vi "Async Test With Results.vi"() -> ()   [LabVIEW 2015, in "ResultProcessor Tests.lvlib"]
uses:
  ResultProcessor Tests.lvlib
  Report Information/DUT Information.ctl
  Report Information/Station Information.ctl
  Report Information/Test Information.ctl
  Execution/ResultProcessor.lvclass
  Config/ResultProcessor Config.lvclass
  Report/On-The-Fly/Config/OnTheFlyReport Config.lvclass
  Report Formatters/csv/Config/csv-formatter Config.lvclass
  Result/Result.lvclass
  Report Information/Report Information.lvclass
panel:
  in  "Report Path":path
  in  "stop":bool
  in  "Measurement":string
  in  "Low Limit":string
  in  "High Limit":string
  in  "Duration (ms)":dbl
  in  "Step Class":string
  in  "Comparison Type":string
  in  "Step Name":string
  in  "Publish Report":bool
  in  "New Report":bool
  in  "Add Result":bool
  in  "Add Test Info":bool
  in  "Add Station Info":bool
  in  "Add DUT Info":bool
  in  "Test Information":T1
  in  "Station Info":T2
  in  "DUT Info":T3
  out "AsyncWorkerError":errorcluster
  out "error out":errorcluster
  # "Run the VI\nPick a file name. Can be an empty file or a new file name.\nSelect New Report\nData entered in the various fields will be sent to the processor each time you press the cooresponding button"
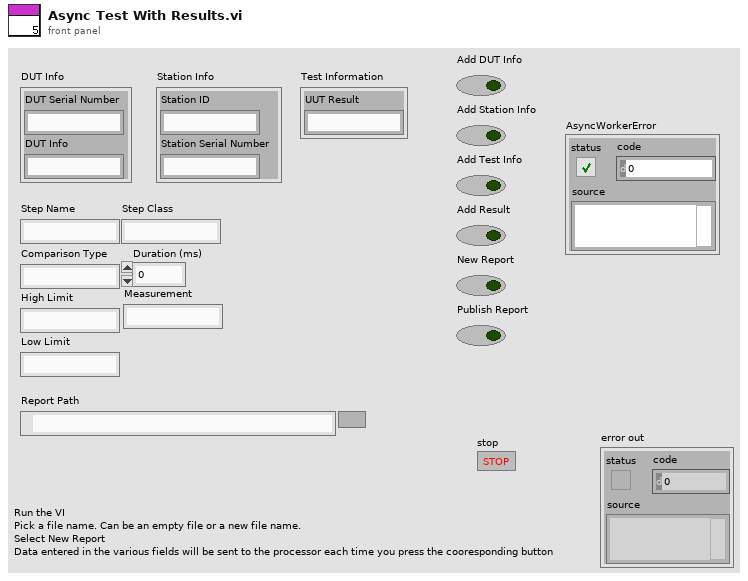
[diagram p1: front panel]
types:
  T1 = typedef "Report Information.lvclass/Test Information.ctl" = cluster{"UUT Result":string}
  T2 = typedef "Report Information.lvclass/Station Information.ctl" = cluster{"Station ID":string, "Station Serial Number":string}
  T3 = typedef "Report Information.lvclass/DUT Information.ctl" = cluster{"DUT Serial Number":string, "DUT Info":string}
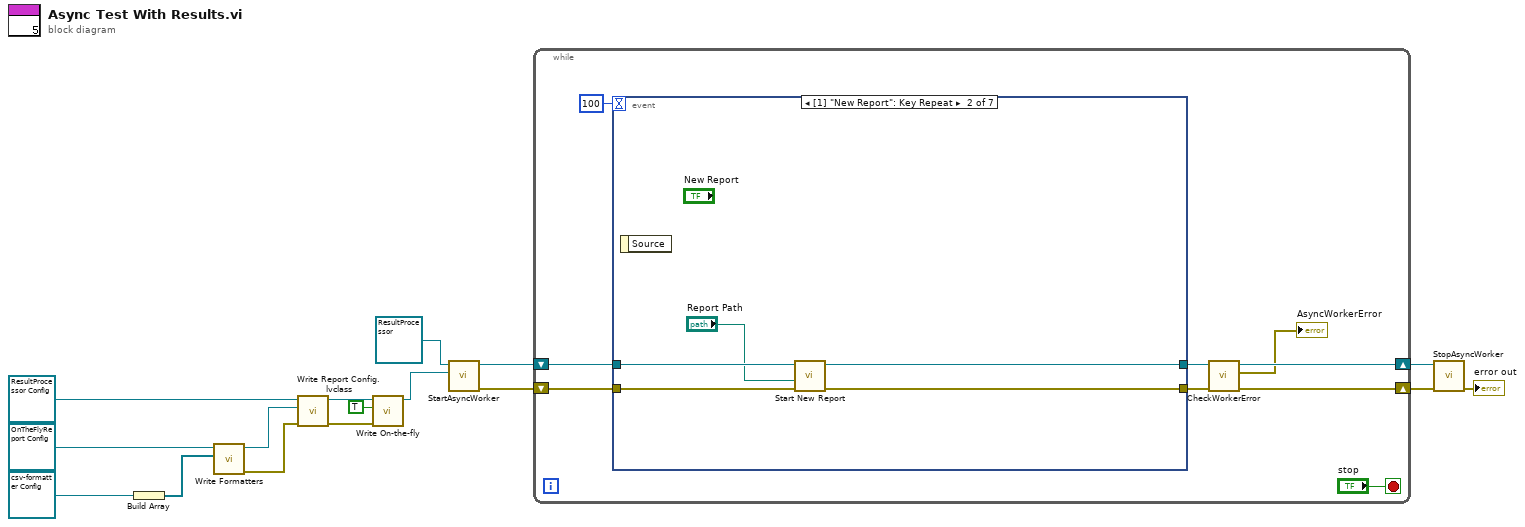
[diagram p0: block diagram]
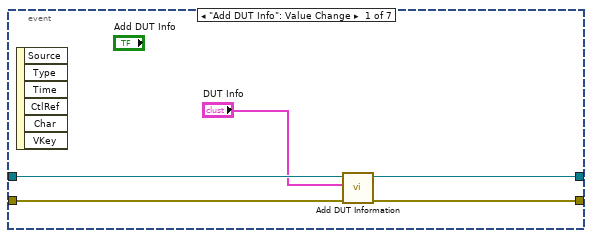
[diagram p2: hidden frame]
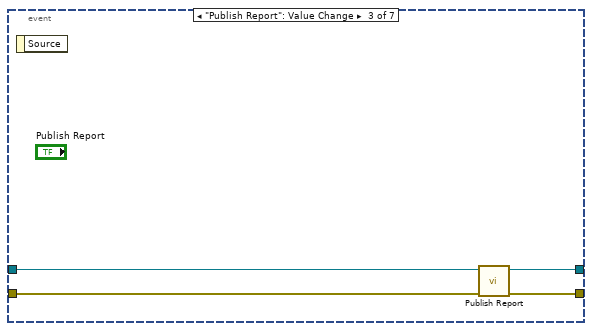
[diagram p3: hidden frame]
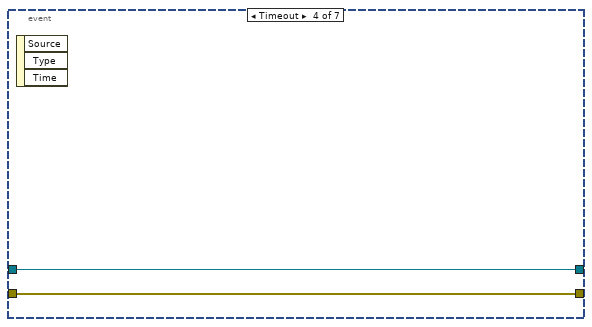
[diagram p4: hidden frame]
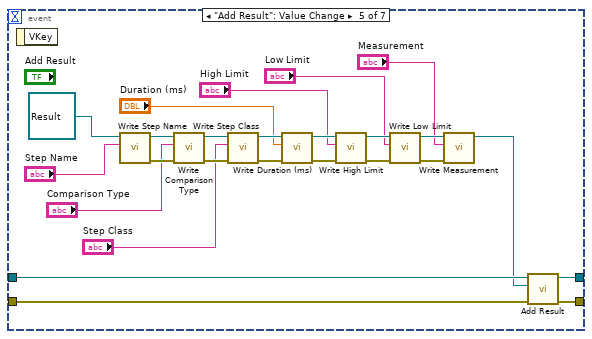
[diagram p5: hidden frame]
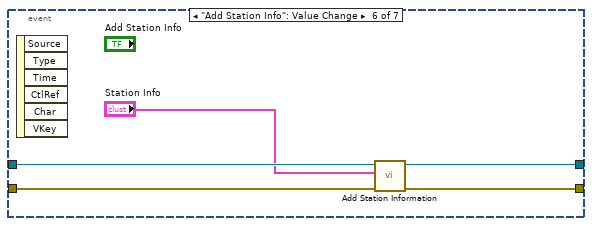
[diagram p6: hidden frame]
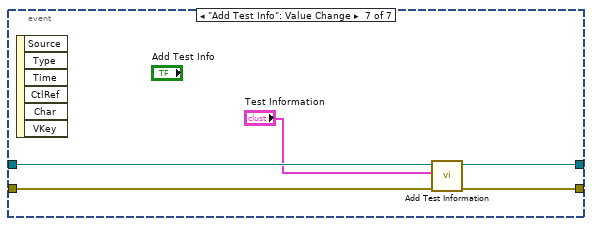
[diagram p7: hidden frame]
diagram:
  n1 = Build Array(refnum<class "csv-formatter Config.lvclass"> refnum ("csv-formatter Config.lvclass")) -> (w6:refnum<class "csv-formatter Config.lvclass">[])
  n2 = call-dynamic "Write Formatters.vi"("Formatters"=w6, "OnTheFlyReport Config in"=refnum<class "OnTheFlyReport Config.lvclass"> refnum ("OnTheFlyReport Config.lvclass")) -> ("error out"=w5:errorcluster, "OnTheFlyReport Config out"=w7:refnum<class "OnTheFlyReport Config.lvclass">)  [unwired: 8 in]
  n3 = call-dynamic "Write Report Config.lvclass.vi"("error in (no error)"=w5, "Report Config.lvclass"=w7, "ResultProcessor Config in"=refnum<class "ResultProcessor Config.lvclass"> refnum) -> ("error out"=w4:errorcluster, "ResultProcessor Config out"=w8:refnum<class "ResultProcessor Config.lvclass">)  [unwired: 7 in]
  n4 = call-dynamic "Write On-the-fly.vi"("error in (no error)"=w4, "On-the-fly?"=TRUE, "ResultProcessor Config in"=w8) -> ("ResultProcessor Config out"=w2:refnum<class "ResultProcessor Config.lvclass">)  [unwired: 7 in, 1 out]
  n5 = call "StartAsyncWorker.vi"("ResultProcessor Config.lvclass"=w2, "ResultProcessor in"=refnum<class "ResultProcessor.lvclass"> refnum ("ResultProcessor.lvclass")) -> ("error out"=w12:errorcluster, "ResultProcessor out"=w15:refnum<class "ResultProcessor.lvclass">)  [unwired: 8 in]
  n6 = while {
    shift-right: [w25] -> w13
    shift-left: w15 -> [w21]
    shift-right: [w24] -> w11
    shift-left: w12 -> [w22]
    stop <- "stop" stop-if-true
    n7 = event shown="[1] \"New Report\": Key Repeat" {
      selector: _ -> [_ _ _ _ _ _ _]
      dyn-events: _ -> [_ _ _ _ _ _ _]
      timeout: 100 -> [_ _ _ _ _ _ _]
      tunnel: w22 -> [w30 w34 w36 w40 w66 w68 w74]
      tunnel: w21 -> [w27 w35 w37 w41 w63 w69 w73]
      tunnel: [w28 w33 w39 w41 w64 w71 w76] -> w20
      tunnel: [w29 w32 w38 w40 w65 w70 w75] -> w19
      event "Add DUT Info": Value Change {
        n8 = event-data() -> ()  [unwired: 1 in, 6 out]
        n9 = call "Add DUT Information.vi"("error in (no error)"=w30, "DUT Info"="DUT Info", "ResultProcessor in"=w27) -> ("error out"=w29:errorcluster, "ResultProcessor out"=w28:refnum<class "ResultProcessor.lvclass">)  [unwired: 7 in]
      }
      event "New Report": Value Change {
        n10 = event-data() -> ()  [unwired: 1 in, 1 out]
        n11 = call "Start New Report.vi"("error in (no error)"=w34, "Report Path"="Report Path", "ResultProcessor in"=w35) -> ("error out"=w32:errorcluster, "ResultProcessor out"=w33:refnum<class "ResultProcessor.lvclass">)  [unwired: 7 in]
      }
      event "Publish Report": Value Change {
        n12 = event-data() -> ()  [unwired: 1 in, 1 out]
        n13 = call "Publish Report.vi"("error in (no error)"=w36, "ResultProcessor in"=w37) -> ("error out"=w38:errorcluster, "ResultProcessor out"=w39:refnum<class "ResultProcessor.lvclass">)  [unwired: 8 in]
      }
      event Timeout {
        n14 = event-data() -> ()  [unwired: 1 in, 3 out]
      }
      event "Add Result": Value Change {
        n15 = event-data() -> ()  [unwired: 1 in, 1 out]
        n16 = call-dynamic "Write Step Name.vi"("Step Name"="Step Name", "Result in"=refnum<class "Result.lvclass"> refnum ("Result.lvclass")) -> ("error out"=w62:errorcluster, "Result out"=w50:refnum<class "Result.lvclass">)  [unwired: 8 in]
        n17 = call-dynamic "Write Comparison Type.vi"("error in (no error)"=w62, "Comparison Type"="Comparison Type", "Result in"=w50) -> ("error out"=w61:errorcluster, "Result out"=w51:refnum<class "Result.lvclass">)  [unwired: 7 in]
        n18 = call-dynamic "Write Step Class.vi"("error in (no error)"=w61, "Step Class"="Step Class", "Result in"=w51) -> ("error out"=w60:errorcluster, "Result out"=w52:refnum<class "Result.lvclass">)  [unwired: 7 in]
        n19 = call-dynamic "Write Duration (ms).vi"("error in (no error)"=w60, "Duration (ms)"="Duration (ms)", "Result in"=w52) -> ("error out"=w59:errorcluster, "Result out"=w53:refnum<class "Result.lvclass">)  [unwired: 7 in]
        n20 = call-dynamic "Write High Limit.vi"("error in (no error)"=w59, "High Limit"="High Limit", "Result in"=w53) -> ("error out"=w58:errorcluster, "Result out"=w54:refnum<class "Result.lvclass">)  [unwired: 7 in]
        n21 = call-dynamic "Write Low Limit.vi"("error in (no error)"=w58, "Low Limit"="Low Limit", "Result in"=w54) -> ("error out"=w57:errorcluster, "Result out"=w55:refnum<class "Result.lvclass">)  [unwired: 7 in]
        n22 = call-dynamic "Write Measurement.vi"("error in (no error)"=w57, "Measurement"="Measurement", "Result in"=w55) -> ("Result out"=w56:refnum<class "Result.lvclass">)  [unwired: 7 in, 1 out]
        n23 = call "Add Result.vi"("error in (no error)"=w66, "Result.lvclass"=w56, "ResultProcessor in"=w63) -> ("error out"=w65:errorcluster, "ResultProcessor out"=w64:refnum<class "ResultProcessor.lvclass">)  [unwired: 7 in]
      }
      event "Add Station Info": Value Change {
        n24 = event-data() -> ()  [unwired: 1 in, 6 out]
        n25 = call "Add Station Information.vi"("error in (no error)"=w68, "Station Info"="Station Info", "ResultProcessor in"=w69) -> ("error out"=w70:errorcluster, "ResultProcessor out"=w71:refnum<class "ResultProcessor.lvclass">)  [unwired: 7 in]
      }
      event "Add Test Info": Value Change {
        n26 = event-data() -> ()  [unwired: 1 in, 6 out]
        n27 = call "Add Test Information.vi"("error in (no error)"=w74, "Test Information"="Test Information", "ResultProcessor in"=w73) -> ("error out"=w75:errorcluster, "ResultProcessor out"=w76:refnum<class "ResultProcessor.lvclass">)  [unwired: 7 in]
      }
    }
    n28 = call "CheckWorkerError.vi"("error in (no error)"=w19, "ResultProcessor in"=w20) -> ("error out"=w24:errorcluster, "AsyncWorkerError"=→"AsyncWorkerError":errorcluster, "ResultProcessor out"=w25:refnum<class "ResultProcessor.lvclass">)  [unwired: 7 in]
  }
  n29 = call "StopAsyncWorker.vi"("error in (no error)"=w11, "ResultProcessor in"=w13) -> ("error out"=→"error out":errorcluster)  [unwired: 8 in, 1 out]
